vi "StringS.vi"(2 "Denominador":dbl[](array[numeric]), 3 "Numerador":dbl[](array[numeric])) -> (0 "String 2":string, 1 "String":string)   [LabVIEW 2020]
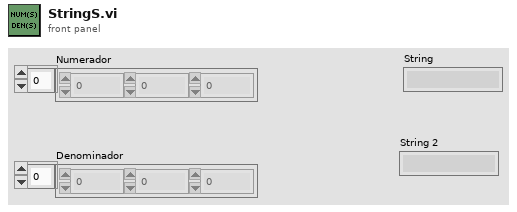
[diagram p1: front panel]
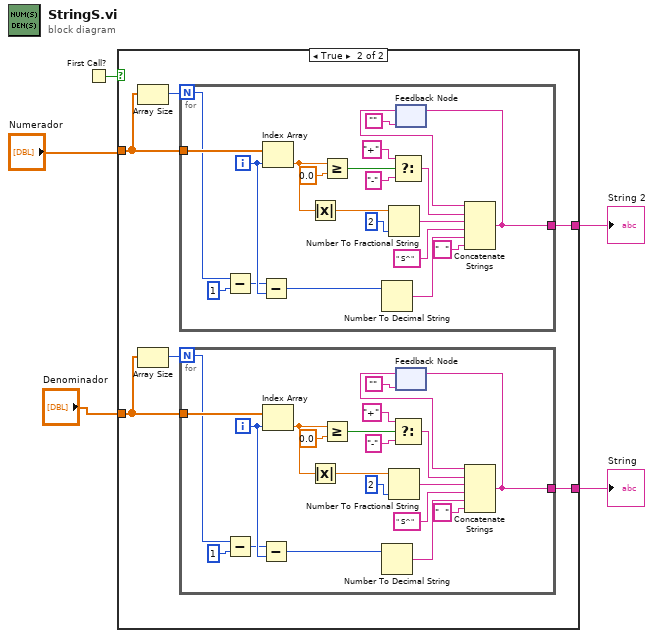
[diagram p0: block diagram]
diagram:
  n1 = First Call?() -> (First Call?: T/F=w5:bool)
  n2 = case shown="True" w5 {
    tunnel: "Denominador" -> [_ w9]
    tunnel: "Numerador" -> [_ w8]
    tunnel: [_ w7] -> w3
    tunnel: [_ w6] -> w4
    frame False {
    }
    frame True {
      n3 = Array Size(array=w8) -> (size(s)=w10:i32)
      n4 = Array Size(array=w9) -> (size(s)=w11:i32)
      n5 = for {
        N: w10 -> [w38]
        tunnel: [w45] -> w7
        tunnel: w8 -> [w40]
        i -> [w44]
        n6 = Subtract(x=w38, y=1) -> (x-y=w37:i32)
        n7 = Subtract(x=w37, y=w44) -> (x-y=w43:i32)
        n8 = Index Array(array=w40, index=w44) -> (element=w39:dbl)
        n9 = Absolute Value(x=w39) -> (abs(x)=w46:dbl)
        n10 = Greater Or Equal?(x=w39, y=0.0) -> (x >= y?=w49:bool)
        n11 = Number To Decimal String(number=w43) -> (decimal integer string=w51:string)  [unwired: 1 in]
        n12 = Number To Fractional String(number=w46, precision (6)=i16 2) -> (F-format string=w52:string)  [unwired: 2 in]
        n13 = Select(t="+", s=w49, f="-") -> (s? t:f=w35:string)
        n14 = feedback #1("") -> (w34:string)
        n15 = Concatenate Strings(w34, w35, w52, " S^", w51, "  " ("string")) -> (w45:string)
        n16 = feedback-in #1(w45) -> ()
      }
      n17 = for {
        N: w11 -> [w17]
        tunnel: [w24] -> w6
        tunnel: w9 -> [w19]
        i -> [w23]
        n18 = Subtract(x=w17, y=1) -> (x-y=w16:i32)
        n19 = Subtract(x=w16, y=w23) -> (x-y=w22:i32)
        n20 = Index Array(array=w19, index=w23) -> (element=w18:dbl)
        n21 = Absolute Value(x=w18) -> (abs(x)=w25:dbl)
        n22 = Greater Or Equal?(x=w18, y=0.0) -> (x >= y?=w28:bool)
        n23 = Number To Decimal String(number=w22) -> (decimal integer string=w30:string)  [unwired: 1 in]
        n24 = Number To Fractional String(number=w25, precision (6)=i16 2) -> (F-format string=w31:string)  [unwired: 2 in]
        n25 = Select(t="+", s=w28, f="-") -> (s? t:f=w14:string)
        n26 = feedback #2("") -> (w13:string)
        n27 = Concatenate Strings(w13, w14, w31, " S^", w30, "  " ("string")) -> (w24:string)
        n28 = feedback-in #2(w24) -> ()
      }
    }
  }
  "String" <- w4
  "String 2" <- w3
